vi "JSON to LVObject - Object with Array of Objects - Returns Object.vi"() -> ()   [LabVIEW 2017, in "Generic Object Serializer Tests.lvlib"]
uses:
  Generic Object Serializer Tests.lvlib
  Generic Object Serializer/Generic Object Serializer.lvclass
  Country/Country.lvclass
  <vilib>/addons/_JKI Toolkits/Caraya/classes/Assert/Assert Equal Value and Type_Variant.vi
  <vilib>/addons/_JKI Toolkits/Caraya/classes/Test/Test.lvclass
  <vilib>/addons/_JKI Toolkits/Caraya/classes/Assert/Assert.lvclass
panel:
  out "error out":errorcluster
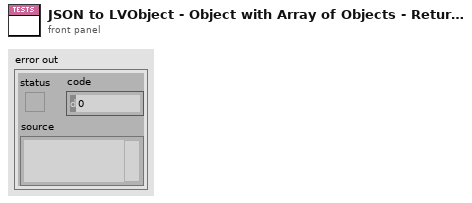
[diagram p1: front panel]
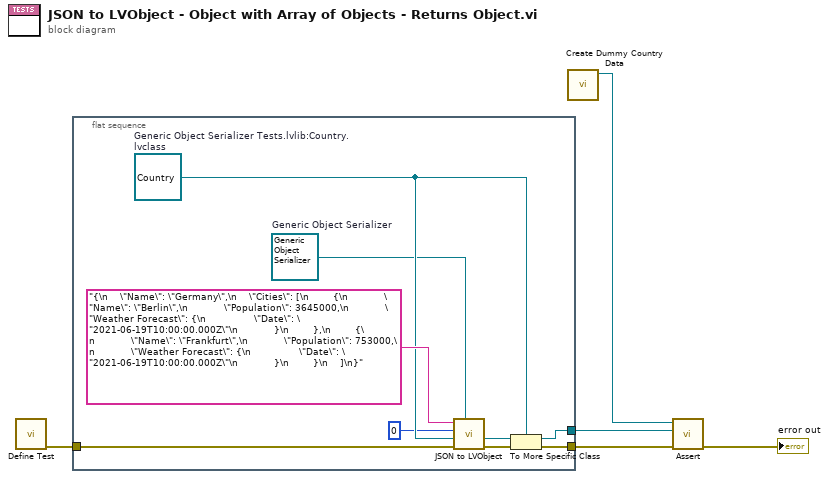
[diagram p0: block diagram]
diagram:
  n1 = call <vilib>:"Define Test.vi"() -> ("error out"=w5:errorcluster)  [unwired: 11 in]
  n2 = flat-sequence {
    tunnel: w5 -> [w8]
    tunnel: [w7] -> w3
    tunnel: [w6] -> w2
    frame #0 {
      w11 = refnum<class "Country.lvclass"> refnum  # Generic Object Serializer Tests.lvlib:Country.lvclass
      w9 = refnum<class "Generic Object Serializer.lvclass"> refnum  # Generic Object Serializer
      n3 = call-dynamic "JSON to LVObject.vi"("LVClass Serializer"=w9, "error in (no error)"=w8, "Object Type"=w11, "Offset"=0, "JSON"="{\n    \"Name\": \"Germany\",\n    \"Cities\": [\n        {\n            \"Name\": \"Berlin\",\n            \"Population\": 3645000,\n            \"Weather Forecast\": {\n                \"Date\": \"2021-06-19T10:00:00.000Z\"\n            }\n        },\n        {\n            \"Name\": \"Frankfurt\",\n            \"Population\": 753000,\n            \"Weather Forecast\": {\n                \"Date\": \"2021-06-19T10:00:00.000Z\"\n            }\n        }\n    ]\n}") -> ("error out"=w14:errorcluster, "Object"=w12:refnum<class>)  [unwired: 5 in]
      n4 = To More Specific Class(target class=w11, reference=w12, error in=w14) -> (specific class reference=w6:refnum<class "Country.lvclass">, error out=w7:errorcluster)
    }
  }
  n5 = call "Create Dummy Country Data.vi"() -> ("Country"=w1:refnum<class "Country.lvclass">)  [unwired: 10 in, 1 out]
  n6 = call-poly <vilib>:"Assert.vi"("error in (no error)"=w3, "Y"=w2, "X"=w1) -> ("error out"=→"error out":errorcluster)  [unwired: 8 in]
